vi "PA_Get.vi"(8 "error in (no error)":errorcluster, 10 "Axis Number":i32, 11 "Agilis in":T1) -> (0 "error out":errorcluster, 2 "Target Position":i32, 3 "Agilis out":T1)   [LabVIEW 2016, in "Drivers.lvlib" / "Agilis.lvlib"]
doc: "Returns current target position."
uses:
  Agilis.lvlib
  AgilisCmdLib Refnum.ctl
  Z:/TraceGrabber/Drivers/Agilis/AgilisCmdLib.dll
  AgilisCmdLib.dll
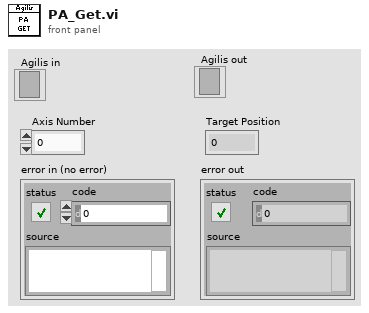
[diagram p1: front panel]
types:
  T1 = typedef "Drivers.lvlib/Agilis.lvlib/AgilisCmdLib Refnum.ctl" = refnum<k24>
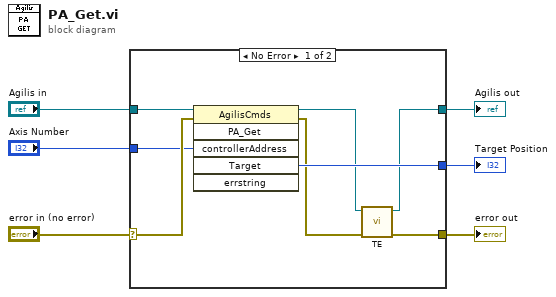
[diagram p0: block diagram]
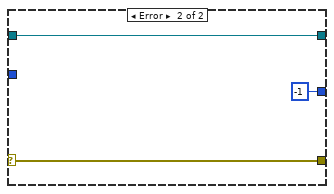
[diagram p2: hidden frame]
diagram:
  n1 = case shown="No Error" "error in (no error)" {
    selector: "error in (no error)" -> [w13 w17]
    tunnel: "Agilis in" -> [w14 w16]
    tunnel: [w7 w16] -> w4
    tunnel: [w10 w17] -> w3
    tunnel: "Axis Number" -> [w12 _]
    tunnel: [w11 -1 ("Target")] -> w1
    frame No Error {
      n2 = invoke class="AgilisCmds" method="PA_Get"(reference=w14, error in=w13, "controllerAddress"=w12) -> (reference out=w8:T1, error out=w9:errorcluster, "Target"=w11:i32)  [unwired: 3 in, 3 out]
      n3 = call "TE.vi"("error in (no error)"=w9, "Agilis in"=w8) -> ("error out"=w10:errorcluster, "Agilis out"=w7:T1)  [unwired: 8 in]
    }
    frame Error {
    }
  }
  "Agilis out" <- w4
  "error out" <- w3
  "Target Position" <- w1
